vi "Get Initial Values.vi"(6 "DISPLAY CHANNEL":i32, 8 "error in":errorcluster, 9 "IMAGE SAVE FORMAT":u32, 10 "String":string, 11 "gRPC ID In":T2) -> (0 "error out":errorcluster)   [LabVIEW 2025, in "Automotive Vision UI.lvlib"]
uses:
  Automotive Vision UI.lvlib
  Automotive-Vision-OOBService_client/Automotive-Vision-OOBService_client.lvlib
  Automotive-Vision-OOBService_client/RPC Messages/hwval_ExportRequest.ctl
  Automotive-Vision-OOBService_client/RPC Messages/hwval_ExportFileType.ctl
  Automotive-Vision-OOBService_client/RPC Messages/hwval_ExportTypeRequest.ctl
  <vilib>/gRPC/LabVIEW gRPC Library/Shared/grpcId.ctl
  <vilib>/gRPC/LabVIEW gRPC Library/grpc-lvsupport-release.lvlib
  Automotive-Vision-OOBService_client/RPC Messages/hwval_GenericRequest.ctl
panel:
  in  "Request Data":T1
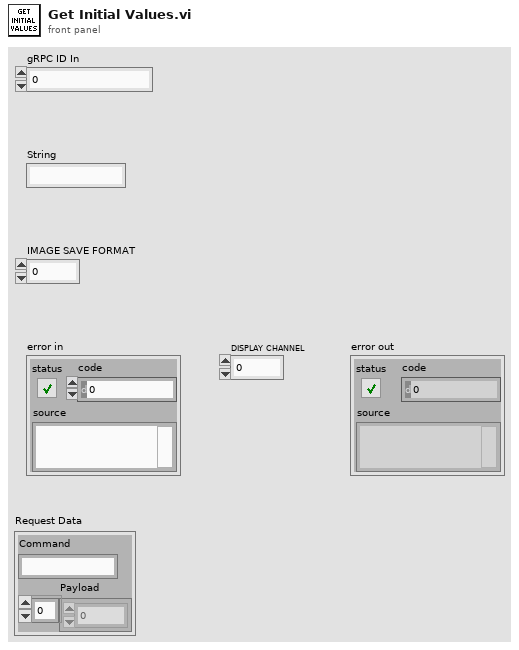
[diagram p1: front panel]
types:
  T1 = typedef "Automotive-Vision-OOBService_client.lvlib/hwval_GenericRequest.ctl" = cluster{"Command":string, "Payload":u8[]}
  T2 = typedef "grpc-lvsupport-release.lvlib/grpcId.ctl" = u64
  T3 = typedef "Automotive-Vision-OOBService_client.lvlib/hwval_ExportTypeRequest.ctl" = cluster{"FileType":T4}
  T4 = typedef "Automotive-Vision-OOBService_client.lvlib/hwval_ExportFileType.ctl" = enum32{"EXPORT_PNG", "EXPORT_RAW"}
  T5 = typedef "Automotive-Vision-OOBService_client.lvlib/hwval_ExportRequest.ctl" = cluster{"FilePath":string}
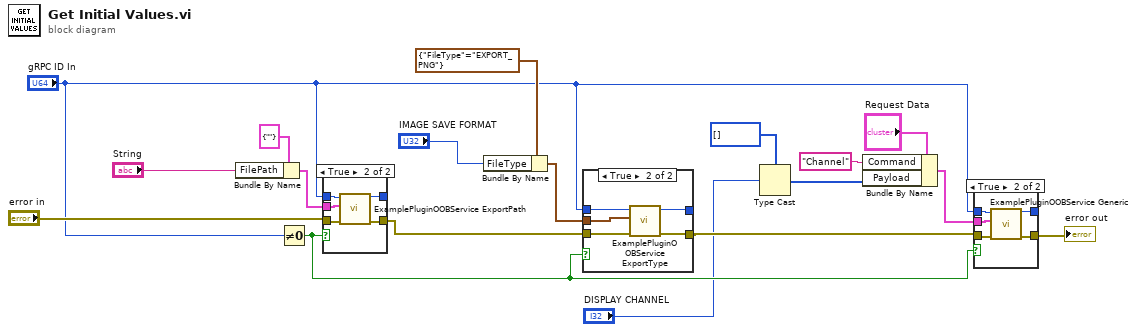
[diagram p0: block diagram]
diagram:
  n1 = Bundle By Name(cluster=T5 {"FilePath"=""} ("Request Data"), "FilePath"="String") -> (w13:T5)
  n2 = Not Equal To 0?(x="gRPC ID In") -> (x != 0?=w9:bool)
  n3 = case shown="True" w9 {
    tunnel: [w20 w24] -> _
    tunnel: [w19 w22] -> w17
    tunnel: "gRPC ID In" -> [w20 w25]
    tunnel: "error in" -> [w19 w23]
    tunnel: w13 -> [_ w21]
    frame False {
    }
    frame True {
      n4 = call "ExamplePluginOOBService ExportPath.vi"("error in"=w23, "Request Data"=w21, "gRPC ID"=w25) -> ("error out"=w22:errorcluster, "gRPC ID out"=w24:T2)  [unwired: 6 in, 1 out]
    }
  }
  n5 = Bundle By Name(cluster=T3 {"FileType"=enum."EXPORT_PNG"} ("Request Data"), "FileType"="IMAGE SAVE FORMAT") -> (w15:T3)
  n6 = case shown="True" w9 {
    tunnel: w17 -> [w26 w30]
    tunnel: [w26 w29] -> w10
    tunnel: "gRPC ID In" -> [w27 w31]
    tunnel: [w27 w28] -> _
    tunnel: w15 -> [_ w32]
    frame False {
    }
    frame True {
      n7 = call "ExamplePluginOOBService ExportType.vi"("error in"=w30, "Request Data"=w32, "gRPC ID"=w31) -> ("error out"=w29:errorcluster, "gRPC ID out"=w28:T2)  [unwired: 6 in, 1 out]
    }
  }
  n8 = Type Cast(type=u8[] [] ("Payload"), x="DISPLAY CHANNEL") -> (*(type *) &x=w4:u8[])
  n9 = Bundle By Name(cluster="Request Data", "Command"="Channel", "Payload"=w4) -> (w2:T1)
  n10 = case shown="True" w9 {
    tunnel: [w34 w38] -> _
    tunnel: [w33 w36] -> w7
    tunnel: "gRPC ID In" -> [w34 w39]
    tunnel: w10 -> [w33 w37]
    tunnel: w2 -> [_ w35]
    frame False {
    }
    frame True {
      n11 = call "ExamplePluginOOBService Generic.vi"("error in"=w37, "Request Data"=w35, "gRPC ID"=w39) -> ("error out"=w36:errorcluster, "gRPC ID out"=w38:T2)  [unwired: 6 in, 1 out]
    }
  }
  "error out" <- w7
